vi "StateMachine.vi"   [LabVIEW 2019]
uses:
  States1.ctl
types:
  T1 = typedef "States1.ctl" = enum16{"Initialize", "Process", "MacroExit", "Exit"}
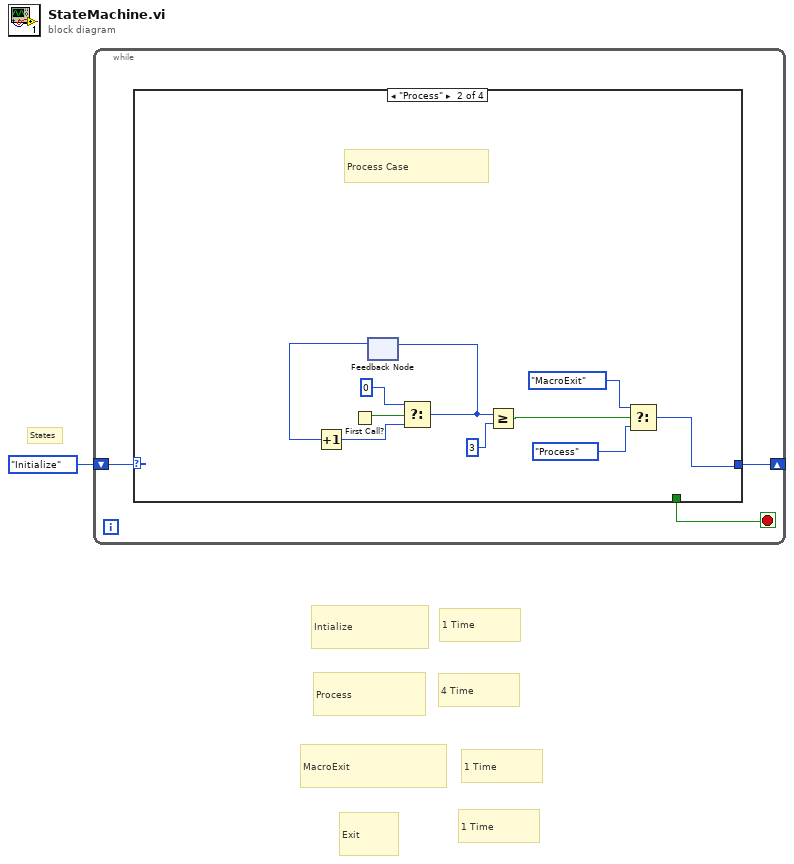
[diagram p0: block diagram]
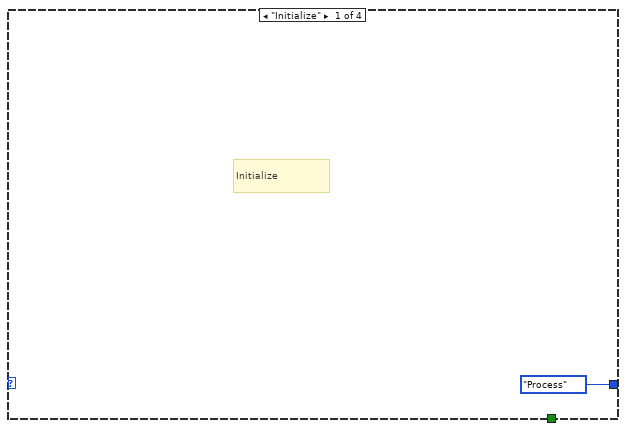
[diagram p2: hidden frame]
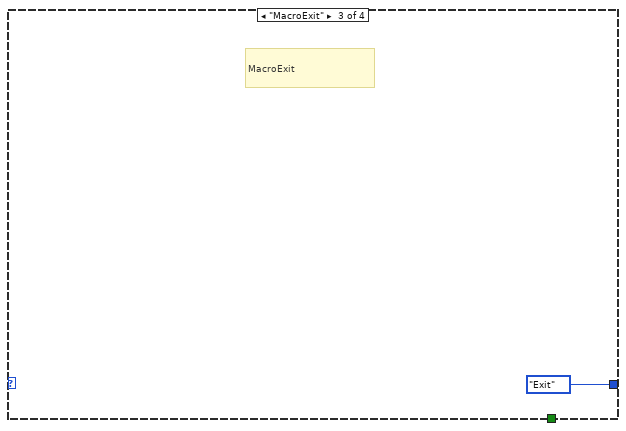
[diagram p3: hidden frame]
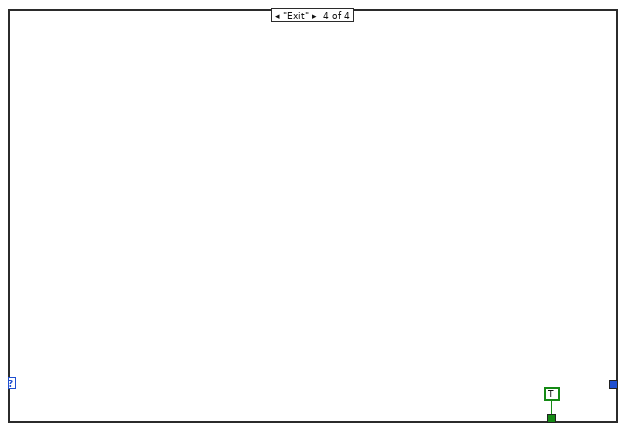
[diagram p4: hidden frame]
diagram:
  # "1 Time"
  # "1 Time"
  # "4 Time"
  # "1 Time"
  # "Exit"
  # "MacroExit"
  # "Process"
  # "Intialize"
  # "States"
  n1 = while {
    shift-right: [w3] -> _
    shift-left: States1."Initialize" -> [w4]
    stop <- w2 stop-if-true
    n2 = case shown="\"Process\"" w4 {
      tunnel: [States1."Process" w6 States1."Exit" _] -> w3
      tunnel: [_ _ _ TRUE] -> w2
      frame "Initialize" {
        # "Initialize"
      }
      frame "Process" {
        # "Process Case"
        n3 = First Call?() -> (First Call?: T/F=w15:bool)
        n4 = feedback #1() -> (w13:i32)  [unwired: 1 in]
        n5 = Increment(x=w13) -> (x+1=w12:i32)
        n6 = Select(t=0, s=w15, f=w12) -> (s? t:f=w11:i32)
        n7 = feedback-in #1(w11) -> ()
        n8 = Greater Or Equal?(x=w11, y=3) -> (x >= y?=w9:bool)
        n9 = Select(t=States1."MacroExit", s=w9, f=States1."Process") -> (s? t:f=w6:T1)
      }
      frame "MacroExit" {
        # "MacroExit"
      }
      frame "Exit" {
      }
    }
  }
